vi "Get Cluster Ring References.vi"(8 "error in (no error)":errorcluster, 11 "Cluster Reference in":refnum<vi>) -> (0 "error out":errorcluster, 3 "Ring References":refnum<vi>[](array[refnum]))   [LabVIEW 2019, in "Control Experiment.lvclass"]
uses:
  <userlib>/LevyLab/Transport/Control Experiment/Control Experiment.lvclass
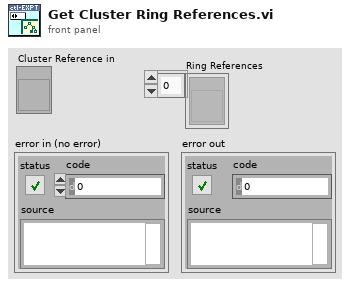
[diagram p1: front panel]
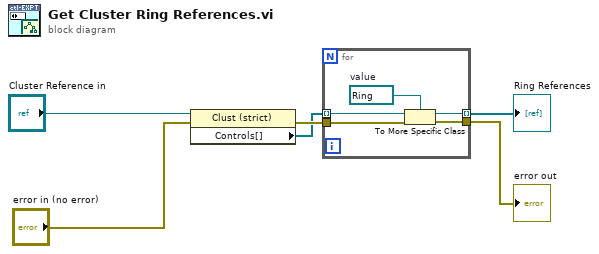
[diagram p0: block diagram]
diagram:
  n1 = property class="Clust (strict)"(reference="Cluster Reference in", error in="error in (no error)") -> (error out=w3:errorcluster, "Controls[]"=w1:refnum<vi>[])  [unwired: 1 out]
  n2 = for {
    tunnel: w1 -> [w10] mode=indexing
    tunnel: [w9] -> w6 mode=indexing
    tunnel: w3 -> [w8]
    tunnel: [w7] -> w2
    w11 = refnum<vi> refnum  # value
    n3 = To More Specific Class(target class=w11, reference=w10, error in=w8) -> (specific class reference=w9:refnum<vi>, error out=w7:errorcluster)
  }
  "Ring References" <- w6
  "error out" <- w2
